vi "Source DC Current4.vi"(8 "error in (no error)":errorcluster, 10 "measurementservice_SMUConfigRequest_Data":T1) -> (0 "error out":errorcluster, 1 "Compliance/Limit Reached":bool, 2 "Current Measurement":sgl, 3 "Voltage Measurement":sgl)   [LabVIEW 2019, in "HVC4.lvlib" / "HVC4.lvclass"]
doc: "Demonstrates how to use the DC Current Output Function to force an output current. This example initializes a session, configures the Output Function, Sense, Autorange, Current Level and Voltage Limit, initiates generation, waits for a specified delay, and measures the voltage and current output. This example uses Single Point source mode."
uses:
  HVC4 Class/HVC4.lvclass
  HVC4 Class/RPC Messages/measurementservice_SMUConfigRequest/measurementservice_SMUConfigRequest_Data.ctl
  <instrlib>/niDCPower/nidcpower.llb/niDCPower Wait For Event - Event.ctl
panel:
  # "Overview: Demonstrates how to use the DC Current Output Function to force an output current.  \nThis example initializes a session, configures the Output Function, Sense, Autorange, Current Level \nand Voltage Limit, initiates generation, waits for a specified delay, and measures the voltage and \ncurrent output.  \nRequirements: NI-DCPower\nInstructions:\n1. Select the appropriate device in the Resource Name control.\n2. Configure the parameters of the DC Current signal you'd like to output.\n3. Run the VI."
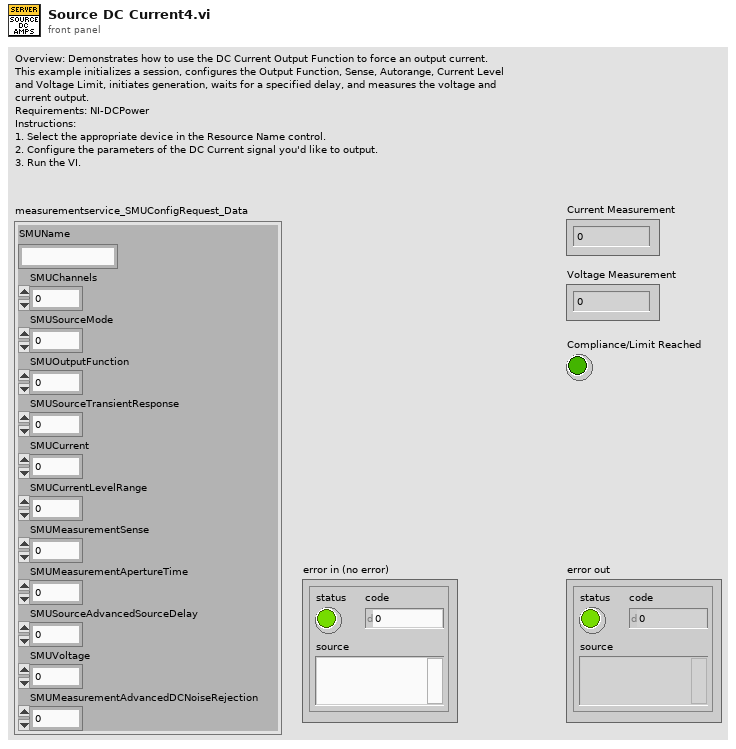
[diagram p1: front panel]
types:
  T1 = typedef "HVC4.lvlib/HVC4.lvclass/measurementservice_SMUConfigRequest_Data.ctl" = cluster{"SMUName":string, "SMUChannels":i32, "SMUSourceMode":i32, "SMUOutputFunction":i32, "SMUSourceTransientResponse":i32, "SMUCurrent":sgl, "SMUCurrentLevelRange":sgl, "SMUMeasurementSense":i32, "SMUMeasurementApertureTime":sgl, "SMUSourceAdvancedSourceDelay":sgl, "SMUVoltage":sgl, "SMUMeasurementAdvancedDCNoiseRejection":i32}
  T2 = typedef "niDCPower Wait For Event - Event.ctl" = i32
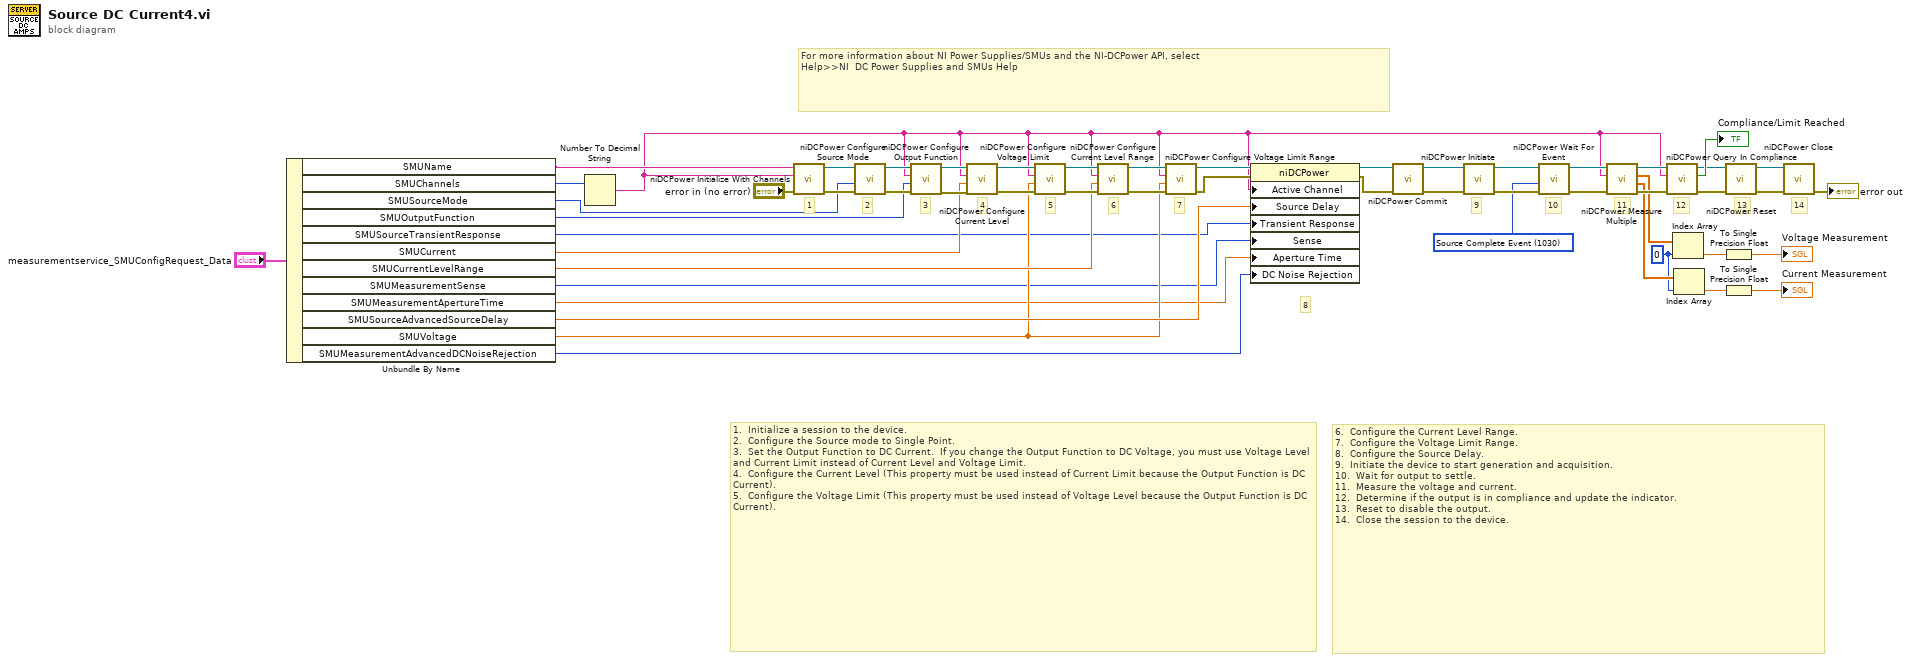
[diagram p0: block diagram]
diagram:
  w10 = T2 1030 items=["Source Complete Event"=1030, "Measure Complete Event"=1031, "Sequence Iteration Complete Event"=1032, "Sequence Engine Done Event"=1033] ("event")
  w15 = 0 ("index")
  # "11"
  # "10"
  # "12"
  # "9"
  # "For more information about NI Power Supplies/SMUs and the NI-DCPower API, select\nHelp>>NI  DC Power Supplies and SMUs Help"
  # "14"
  # "8"
  # "7"
  # "6"
  # "2"
  # "1.  Initialize a session to the device.\n2.  Configure the Source mode to Single Point.\n3.  Set the Output Function to DC Current.  If you change the Output Function to DC Voltage, you must use Voltage Level and Current Limit instead of Current Level and Voltage Limit.\n4.  Configure the Current Level (This property must be used instead of Current Limit because the Output Function is DC Current).\n5.  Configure the Voltage Limit (This property must be used instead of Voltage Level because the Output Function is DC Current)."
  # "3"
  # "6.  Configure the Current Level Range.\n7.  Configure the Voltage Limit Range.\n8.  Configure the Source Delay.\n9.  Initiate the device to start generation and acquisition.\n10.  Wait for output to settle.\n11.  Measure the voltage and current.\n12.  Determine if the output is in compliance and update the indicator.\n13.  Reset to disable the output.\n14.  Close the session to the device."
  # "13"
  # "5"
  # "4"
  # "1"
  n1 = Unbundle By Name("measurementservice_SMUConfigRequest_Data") -> ("SMUName"=w22:string, "SMUChannels"=w34:i32, "SMUSourceMode"=w33:i32, "SMUOutputFunction"=w32:i32, "SMUSourceTransientResponse"=w27:i32, "SMUCurrent"=w31:sgl, "SMUCurrentLevelRange"=w30:sgl, "SMUMeasurementSense"=w26:i32, "SMUMeasurementApertureTime"=w25:sgl, "SMUSourceAdvancedSourceDelay"=w29:sgl, "SMUVoltage"=w28:sgl, "SMUMeasurementAdvancedDCNoiseRejection"=w24:i32)
  n2 = Number To Decimal String(number=w34) -> (decimal integer string=w7:string)  [unwired: 1 in]
  n3 = call <instrlib>:"niDCPower Initialize With Channels.vi"("error in (no error)"="error in (no error)", "channels"=w7, "resource name"=w22) -> ("error out"=w48:errorcluster, "instrument handle out"=w47:refnum<k15>)  [unwired: 2 in, 5 out]
  n4 = call <instrlib>:"niDCPower Configure Source Mode.vi"("error in (no error)"=w48, "source mode"=w33, "instrument handle"=w47) -> ("error out"=w46:errorcluster, "instrument handle out"=w45:refnum<k15>)  [unwired: 7 out]
  n5 = call <instrlib>:"niDCPower Configure Output Function.vi"("error in (no error)"=w46, "output function"=w32, "channel name"=w7, "instrument handle"=w45) -> ("error out"=w38:errorcluster, "instrument handle out"=w37:refnum<k15>)  [unwired: 6 out]
  n6 = call <instrlib>:"niDCPower Configure Current Level.vi"("error in (no error)"=w38, "current level"=w31, "channel name"=w7, "instrument handle"=w37) -> ("error out"=w52:errorcluster, "instrument handle out"=w53:refnum<k15>)  [unwired: 6 out]
  n7 = call <instrlib>:"niDCPower Configure Voltage Limit.vi"("error in (no error)"=w52, "voltage limit"=w28, "channel name"=w7, "instrument handle"=w53) -> ("error out"=w44:errorcluster, "instrument handle out"=w43:refnum<k15>)  [unwired: 6 out]
  n8 = call <instrlib>:"niDCPower Configure Current Level Range.vi"("error in (no error)"=w44, "current level range"=w30, "channel name"=w7, "instrument handle"=w43) -> ("error out"=w42:errorcluster, "instrument handle out"=w41:refnum<k15>)  [unwired: 6 out]
  n9 = call <instrlib>:"niDCPower Configure Voltage Limit Range.vi"("error in (no error)"=w42, "voltage limit range"=w28, "channel name"=w7, "instrument handle"=w41) -> ("error out"=w39:errorcluster, "instrument handle out"=w40:refnum<k15>)  [unwired: 6 out]
  n10 = property class="niDCPower"(reference=w40, error in=w39, "Active Channel"=w7, "Source Delay"=w29, "Transient Response"=w27, "Sense"=w26, "Aperture Time"=w25, "DC Noise Rejection"=w24) -> (reference out=w36:refnum<k15>, error out=w35:errorcluster)
  n11 = call <instrlib>:"niDCPower Commit.vi"("error in (no error)"=w35, "instrument handle"=w36) -> ("error out"=w8:errorcluster, "instrument handle out"=w9:refnum<k15>)  [unwired: 8 in]
  n12 = call <instrlib>:"niDCPower Initiate.vi"("error in (no error)"=w8, "instrument handle"=w9) -> ("error out"=w12:errorcluster, "instrument handle out"=w14:refnum<k15>)  [unwired: 2 in, 6 out]
  n13 = call <instrlib>:"niDCPower Wait For Event.vi"("error in (no error)"=w12, "event"=w10, "instrument handle"=w14) -> ("error out"=w11:errorcluster, "instrument handle out"=w13:refnum<k15>)  [unwired: 1 in, 6 out]
  n14 = call <instrlib>:"niDCPower Measure Multiple.vi"("error in (no error)"=w11, "channel name"=w7, "instrument handle"=w13) -> ("error out"=w19:errorcluster, "current measurements"=w16:dbl[], "voltage measurements"=w17:dbl[], "instrument handle out"=w20:refnum<k15>)  [unwired: 5 out]
  n15 = call <instrlib>:"niDCPower Query In Compliance.vi"("error in (no error)"=w19, "channel name"=w7, "instrument handle"=w20) -> ("error out"=w5:errorcluster, "in compliance?"=→"Compliance/Limit Reached":bool, "instrument handle out"=w6:refnum<k15>)  [unwired: 6 out]
  n16 = Index Array(array=w17, index=w15) -> (element=w4:dbl)
  n17 = Index Array(array=w16, index=w15) -> (element=w2:dbl)
  n18 = To Single Precision Float(number=w4) -> (single precision float=→"Voltage Measurement":sgl)
  n19 = To Single Precision Float(number=w2) -> (single precision float=→"Current Measurement":sgl)
  n20 = call <instrlib>:"niDCPower Reset.vi"("error in (no error)"=w5, "instrument handle"=w6) -> ("error out"=w50:errorcluster, "instrument handle out"=w51:refnum<k15>)  [unwired: 2 in, 6 out]
  n21 = call <instrlib>:"niDCPower Close.vi"("error in (no error)"=w50, "instrument handle"=w51) -> ("error out"=→"error out":errorcluster)  [unwired: 9 out]
